vi "Lab Panel V6.00.vi"() -> ()   [LabVIEW 2017] (continued)
                    n2891 = local read "SIG LAB04-2"() -> (w5335:T2)
                    n2892 = local read "RESULT LAB04-2"() -> (w5322:bool)
                    n2893 = Bundle("FAIL LAB04-2"=w5325, "SIG LAB04-2"=w5335, "TEMP START LAB04-2"=w5334, "DISP LAB04-2"=w5331, "SET LAB04-2"=w5330, "TDMS LAB04-2"=w5333) -> (w5320:T47)  [unwired: 1 in]
                    n2894 = call "sub vi - cycle&temp fail v7.vi"("Amps Lo?"=w5332, "Input Cluster"=w5320, "SELECT"=w5329, "Amps Hi?"=w5328, "Result In"=w5322, "Panel"=u64 8) -> ("(FAIL) out"=w5324:cluster{"FAIL LO":dbl, "FAIL HI":dbl}, "(DISP) out"=w5327:T40, "T-RISE"=w5321:cluster{"T-RISE (L)":dbl, "T-RISE (N)":dbl}, "Result Out"=w5323:bool, "file error"=w5326:errorcluster)  [unwired: 9 in]
                    n2895 = local write "TEMP RISE LAB04-2"(w5321) -> ()
                    n2896 = local write "FAIL LAB04-2"(w5324) -> ()
                    n2897 = local write "DISP LAB04-2"(w5327) -> ()
                    n2898 = local write "RESULT LAB04-2"(w5323) -> ()
                    n2899 = local write "data file error"(w5326) -> ()
                  }
                }
              }
              frame #8 {
                # "LAB05-1"
                n2900 = Index Array(array=w5338, index=4) -> (element=w5341:bool)
                n2901 = Not(x=w5341) -> (.not. x?=w5339:bool)
                n2902 = And(x=w5339, y=w5337) -> (x .and. y?=w5336:bool)
                n2903 = case shown="True" w5336 {
                  tunnel: w5344 -> [_ w5358]
                  tunnel: w5342 -> [_ w5355]
                  tunnel: w5343 -> [_ w5354]
                  frame False {
                  }
                  frame True {
                    n2904 = local read "TEMP START LAB05-1"() -> (w5360:cluster{"TL":dbl, "TN":dbl})
                    n2905 = local read "FAIL LAB05-1"() -> (w5351:cluster{"LO":dbl, "HI":dbl})
                    n2906 = local read "TDMS LAB05-1"() -> (w5359:refnum<k34>)
                    n2907 = local read "SET LAB05-1"() -> (w5356:T5)
                    n2908 = local read "DISP LAB05-1"() -> (w5357:T4)
                    n2909 = local read "SIG LAB05-1"() -> (w5361:T2)
                    n2910 = local read "RESULT LAB05-1"() -> (w5348:bool)
                    n2911 = Bundle("FAIL LAB05-1"=w5351, "SIG LAB05-1"=w5361, "TEMP START LAB05-1"=w5360, "DISP LAB05-1"=w5357, "SET LAB05-1"=w5356, "TDMS LAB05-1"=w5359) -> (w5346:T48)  [unwired: 1 in]
                    n2912 = call "sub vi - cycle&temp fail v7.vi"("Amps Lo?"=w5358, "Input Cluster"=w5346, "SELECT"=w5355, "Amps Hi?"=w5354, "Result In"=w5348, "Panel"=u64 9) -> ("(FAIL) out"=w5350:cluster{"FAIL LO":dbl, "FAIL HI":dbl}, "(DISP) out"=w5353:T40, "T-RISE"=w5347:cluster{"T-RISE (L)":dbl, "T-RISE (N)":dbl}, "Result Out"=w5349:bool, "file error"=w5352:errorcluster)  [unwired: 9 in]
                    n2913 = local write "TEMP RISE LAB05-1"(w5347) -> ()
                    n2914 = local write "FAIL LAB05-1"(w5350) -> ()
                    n2915 = local write "DISP LAB05-1"(w5353) -> ()
                    n2916 = local write "RESULT LAB05-1"(w5349) -> ()
                    n2917 = local write "data file error"(w5352) -> ()
                  }
                }
              }
              frame #9 {
                # "LAB05-2"
                n2918 = Index Array(array=w5364, index=4) -> (element=w5367:bool)
                n2919 = Not(x=w5367) -> (.not. x?=w5365:bool)
                n2920 = And(x=w5365, y=w5363) -> (x .and. y?=w5362:bool)
                n2921 = case shown="True" w5362 {
                  tunnel: w5370 -> [_ w5384]
                  tunnel: w5368 -> [_ w5381]
                  tunnel: w5369 -> [_ w5380]
                  frame False {
                  }
                  frame True {
                    n2922 = local read "TEMP START LAB05-2"() -> (w5386:cluster{"TL":dbl, "TN":dbl})
                    n2923 = local read "FAIL LAB05-2"() -> (w5377:cluster{"LO":dbl, "HI":dbl})
                    n2924 = local read "TDMS LAB05-2"() -> (w5385:refnum<k34>)
                    n2925 = local read "SET LAB05-2"() -> (w5382:T5)
                    n2926 = local read "DISP LAB05-2"() -> (w5383:T4)
                    n2927 = local read "SIG LAB05-2"() -> (w5387:T2)
                    n2928 = local read "RESULT LAB05-2"() -> (w5374:bool)
                    n2929 = Bundle("FAIL LAB05-2"=w5377, "SIG LAB05-2"=w5387, "TEMP START LAB05-2"=w5386, "DISP LAB05-2"=w5383, "SET LAB05-2"=w5382, "TDMS LAB05-2"=w5385) -> (w5372:T49)  [unwired: 1 in]
                    n2930 = call "sub vi - cycle&temp fail v7.vi"("Amps Lo?"=w5384, "Input Cluster"=w5372, "SELECT"=w5381, "Amps Hi?"=w5380, "Result In"=w5374, "Panel"=u64 10) -> ("(FAIL) out"=w5376:cluster{"FAIL LO":dbl, "FAIL HI":dbl}, "(DISP) out"=w5379:T40, "T-RISE"=w5373:cluster{"T-RISE (L)":dbl, "T-RISE (N)":dbl}, "Result Out"=w5375:bool, "file error"=w5378:errorcluster)  [unwired: 9 in]
                    n2931 = local write "TEMP RISE LAB05-2"(w5373) -> ()
                    n2932 = local write "FAIL LAB05-2"(w5376) -> ()
                    n2933 = local write "DISP LAB05-2"(w5379) -> ()
                    n2934 = local write "RESULT LAB05-2"(w5375) -> ()
                    n2935 = local write "data file error"(w5378) -> ()
                  }
                }
              }
            }
            n2936 = global write "Global 1.vi" "fail count"(w5101) -> ()
          }
          frame #17 {
            # "run calibration routine"
            n2937 = case shown="True" "SET (cal)" {
              frame False {
              }
              frame True {
                n2938 = stacked-sequence {
                  seq-local: [w5389 _ _] -> [_ w5391 _]
                  frame #0 {
                    n2939 = call "CALIBRATION PASSWORD"() -> ("PASSWORD"=w5389:string)  [unwired: 17 in, 2 out]
                  }
                  frame #1 {
                    n2940 = Equal?(x=w5391, y="7777") -> (x = y?=w5390:bool)
                    n2941 = case shown="True" w5390 {
                      frame False {
                      }
                      frame True {
                        n2942 = stacked-sequence {
                          frame #0 {
                            n2943 = local read "SAMPLES"() -> (w5393:dbl)
                            n2944 = local read "AI Task2"() -> (w5394:u32)
                            n2945 = local read "AI Task1"() -> (w5395:u32)
                            n2946 = local read "AI Task0"() -> (w5396:u64)
                            n2947 = local read "Temp Test Cal"() -> (w5397:dbl)
                            n2948 = call "sub vi - calibration v2.vi"("Samples"=w5393, "Task2"=w5394, "Task1"=w5395, "Task0"=w5396, "Temp Test Cal"=w5397) -> ()  [unwired: 7 in]
                          }
                          frame #1 {
                            n2949 = call "sub vi - get calibration values v1.vi"() -> ("TEMP REF CAL"=w5399:dbl, "LAB01 (CAL)"=w5403:T15, "LAB02 (CAL)"=w5402:T16, "LAB03 (CAL)"=w5401:T15, "LAB04 (CAL)"=w5400:T15, "calibration file error out"=w5404:errorcluster, "LAB05 (CAL)"=w5398:T15)  [unwired: 9 in]
                            n2950 = local write "TEMP REF cal"(w5399) -> ()
                            n2951 = local write "cal file error out"(w5404) -> ()
                            n2952 = local write "CAL LAB04"(w5400) -> ()
                            n2953 = local write "LAB05 (CAL)"(w5398) -> ()
                            n2954 = local write "CAL LAB01"(w5403) -> ()
                            n2955 = local write "CAL LAB02"(w5402) -> ()
                            n2956 = local write "CAL LAB03"(w5401) -> ()
                          }
                        }
                      }
                    }
                  }
                  frame #2 {
                    n2957 = local write "SET (cal)"(FALSE) -> ()
                  }
                }
              }
            }
          }
          frame #18 {
            # "save certain settings to file"
            n2958 = String To Path(string="c:\\crabtree\\Set Up\\") -> (path=w5407:path)
            n2959 = Build Path(base path=w5407, name or relative path="settings.bin") -> (appended path=w5409:path)
            n2960 = Build Path(base path=w5407, name or relative path="mail.bin") -> (appended path=w5406:path)
            n2961 = Create Folder(path (use dialog)=w5407) -> (error out=w5412:errorcluster)  [unwired: 2 in, 2 out]
            n2962 = call <vilib>:"Clear Errors.vi"("error in (no error)"=w5412) -> ()  [unwired: 5 in, 2 out]
            n2963 = stacked-sequence {
              seq-local: [w5426 _] -> [_ w5439]
              tunnel: w5409 -> [_ w5440]
              tunnel: w5406 -> [_ w5438]
              frame #0 {
                n2964 = local read "Set Loop Time"() -> (w5414:T14)
                n2965 = local read "DigOutDelay"() -> (w5413:u32)
                n2966 = local read "Network Directory"() -> (w5431:path)
                n2967 = local read "C drive data root dir"() -> (w5425:path)
                n2968 = local read "RATE (Hz)"() -> (w5424:dbl)
                n2969 = local read "SAMPLES"() -> (w5423:dbl)
                n2970 = local read "Select COM port"() -> (w5422:refnum<visa-resource-name>)
                n2971 = local read "Temp Delay Lps"() -> (w5421:dbl)
                n2972 = local read "Temp Value"() -> (w5420:dbl)
                n2973 = local read "Fail Loops"() -> (w5419:dbl)
                n2974 = local read "Temp Test Cal"() -> (w5418:dbl)
                n2975 = local read "Amps Fail level"() -> (w5417:dbl)
                n2976 = local read "Mail Test File To:"() -> (w5416:string)
                n2977 = local read "Mail Test Fail"() -> (w5415:bool)
                n2978 = local read "SET LAB05-2"() -> (w5430:T5)
                n2979 = local read "SET LAB05-1"() -> (w5429:T5)
                n2980 = local read "SET LAB04-2"() -> (w5428:T5)
                n2981 = local read "SET LAB03-2"() -> (w5432:T5)
                n2982 = local read "SET LAB04-1"() -> (w5427:T5)
                n2983 = local read "SET LAB03-1"() -> (w5433:T5)
                n2984 = local read "SET LAB02-2"() -> (w5434:T5)
                n2985 = local read "SET LAB02-1"() -> (w5435:T5)
                n2986 = local read "SET LAB01-2"() -> (w5436:T5)
                n2987 = local read "SET LAB01-1"() -> (w5437:T5)
                n2988 = Bundle("SET LAB01-1"=w5437, "SET LAB01-2"=w5436, "SET LAB02-1"=w5435, "SET LAB02-2"=w5434, "SET LAB03-1"=w5433, "SET LAB03-2"=w5432, "SET LAB04-1"=w5427, "SET LAB04-2"=w5428, "SET LAB05-1"=w5429, "SET LAB05-2"=w5430, "Network Directory"=w5431, "C drive data root dir"=w5425, "RATE (Hz)"=w5424, "SAMPLES"=w5423, "Select COM port"=w5422, "Temp Delay Lps"=w5421, "Temp Value"=w5420, "Fail Loops"=w5419, "Temp Test Cal"=w5418, "Amps Fail level"=w5417, "Mail Test File To:"=w5416, "Mail Test Fail"=w5415, "Set Loop Time"=w5414, "DigOutDelay"=w5413) -> (w5426:T26)  [unwired: 1 in]
              }
              frame #1 {
                n2989 = event shown="[1] \"SET LAB01-1\", \"SET LAB01-2\", \"SET LAB02-1\", \"SET LAB02-2\", \"SET LAB03-1\", \"SET LAB03-2\", \"SET LAB04-1\", \"SET LAB04-2\", \"SET LAB05-1\", \"SET LAB05-2\", \"Network Directory\", \"C drive data root dir\", \"RATE (Hz)\", \"SAMPLES\", \"Select COM port\", \"Temp Delay Lps\", \"Temp Value\", \"Fail Loops\", \"Temp Test Cal\", \"Amps Fail level\", \"Mail Test File To:\", \"Mail Test Fail\", \"Set Loop Time\", \"DigOutDelay\": Value Change" {
                  selector: _ -> [_ _ _]
                  dyn-events: _ -> [_ _ _]
                  timeout: 0.0 -> [_ _ _]
                  tunnel: w5440 -> [_ w5442 _]
                  tunnel: w5439 -> [_ w5443 _]
                  tunnel: w5438 -> [_ _ w5454]
                  event Timeout {
                    n2990 = event-data() -> ()  [unwired: 1 in, 3 out]
                  }
                  event "Network Directory", "C drive data root dir", "RATE (Hz)", "SAMPLES", "Select COM port", "Temp Delay Lps", "Temp Value", "Fail Loops", "Temp Test Cal", "Amps Fail level", "Mail Test File To:", "Mail Test Fail", "DigOutDelay": Value Change {
                    # "Write Settings File"
                    n2991 = event-data() -> ()  [unwired: 1 in, 6 out]
                    n2992 = Open/Create/Replace File(file path (use dialog)=w5442, operation (0:open)=T19."replace or create") -> (refnum out=w5448:refnum<file>, error out=w5447:errorcluster)  [unwired: 4 in, 1 out]
                    n2993 = Write to Binary File(file (use dialog)=w5448, data=w5443, error in=w5447) -> (refnum out=w5446:refnum<file>, error out=w5445:errorcluster)  [unwired: 3 in, 1 out]
                    n2994 = Close File(refnum=w5446, error in=w5445) -> (error out=w5444:errorcluster)  [unwired: 1 out]
                    n2995 = local write "data file error"(w5444) -> ()
                  }
                  event "MAIL SETTINGS.OUT SERVER ADDRESS", "MAIL SETTINGS.FROM ACCOUNT", "MAIL SETTINGS.USER NAME", "MAIL SETTINGS.PASSWORD", "Auto Mail Send", "TO (string):": Value Change {
                    n2996 = event-data() -> ()  [unwired: 1 in, 6 out]
                    n2997 = local read "Auto Mail Send"() -> (w5451:bool)
                    n2998 = local read "MAIL SETTINGS"() -> (w5453:T7)
                    n2999 = local read "TO (string):"() -> (w5450:string)
                    n3000 = Open/Create/Replace File(file path (use dialog)=w5454, operation (0:open)=T19."replace or create") -> (refnum out=w5459:refnum<file>, error out=w5458:errorcluster)  [unwired: 4 in, 1 out]
                    n3001 = Bundle("MAIL SETTINGS"=w5453, "Auto Mail Send"=w5451, "TO (string):"=w5450) -> (w5452:T50)  [unwired: 1 in]
                    n3002 = Write to Binary File(file (use dialog)=w5459, data=w5452, error in=w5458) -> (refnum out=w5457:refnum<file>, error out=w5456:errorcluster)  [unwired: 3 in, 1 out]
                    n3003 = Close File(refnum=w5457, error in=w5456) -> (error out=w5455:errorcluster)  [unwired: 1 out]
                    n3004 = local write "data file error"(w5455) -> ()
                  }
                }
              }
            }
          }
          frame #19 {
            # "mail control"
            n3005 = local read "MAIL SETTINGS"() -> (w5476:T7)
            n3006 = local read "Auto Mail Send"() -> (w5462:bool)
            n3007 = Unbundle By Name(w5476) -> ("OUT SERVER ADDRESS"=w5475:string, "FROM ACCOUNT"=w5474:string, "TEST MAIL"=w5473:bool)
            n3008 = stacked-sequence {
              tunnel: "TO (string):" -> [_ w5515]
              tunnel: w5476 -> [w5481 w5514]
              tunnel: w5475 -> [w5480 w5513]
              tunnel: w5474 -> [w5479 w5512]
              tunnel: w5473 -> [w5478 _]
              tunnel: w5462 -> [_ w5511]
              tunnel: w5472 -> [_ w5510]
              tunnel: w5471 -> [_ w5509]
              tunnel: w5470 -> [_ w5508]
              tunnel: w5469 -> [_ w5507]
              tunnel: w5468 -> [_ w5506]
              tunnel: w5467 -> [_ w5505]
              tunnel: w5466 -> [_ w5504]
              tunnel: w5465 -> [_ w5503]
              tunnel: w5464 -> [_ w5502]
              tunnel: w5463 -> [_ w5501]
              tunnel: "TO (string):" -> [w5477 _]
              frame #0 {
                # "mail test"
                n3009 = case shown="True" w5478 {
                  tunnel: w5481 -> [_ w5485]
                  tunnel: w5477 -> [_ w5484]
                  tunnel: w5480 -> [_ w5483]
                  tunnel: w5479 -> [_ w5482]
                  frame False {
                  }
                  frame True {
                    n3010 = stacked-sequence {
                      seq-local: [_ _ w5495 _] -> [_ _ _ w5496]
                      tunnel: w5485 -> [w5488 _ _ w5500]
                      tunnel: w5484 -> [_ _ w5493 _]
                      tunnel: w5483 -> [_ _ w5491 _]
                      tunnel: w5482 -> [_ _ w5492 _]
                      frame #0 {
                        n3011 = Bundle(cluster=w5488, "TEST MAIL STATUS"="TEST START") -> (w5486:T7)  [unwired: 6 in]
                        n3012 = local write "MAIL SETTINGS"(w5486) -> ()
                      }
                      frame #1 {
                        n3013 = Wait (ms)(milliseconds to wait=500) -> ()  [unwired: 1 out]
                      }
                      frame #2 {
                        n3014 = call "Lab Send Mail Test.vi"("TO:"=w5493, "subject"="MAIL TEST FROM LAB PANEL", "from"=w5492, "out going server"=w5491, "message"="TEST MESSAGE") -> ("error out"=w5495:errorcluster)  [unwired: 10 in]
                      }
                      frame #3 {
                        n3015 = Bundle(cluster=w5500, "TEST MAIL"=FALSE, "TEST MAIL STATUS"="TEST END", "mail error"=w5496) -> (w5498:T7)  [unwired: 4 in]
                        n3016 = local write "MAIL SETTINGS"(w5498) -> ()
                      }
                    }
                  }
                }
              }
              frame #1 {
                # "mail report"
                n3017 = stacked-sequence {
                  seq-local: [_ w5558 _ _] -> [_ _ _ w5748]
                  seq-local: [_ _ w5661 _] -> [_ _ _ w5738]
                  seq-local: [w5525 _ _ _] -> [_ w5575 _ _]
                  seq-local: [w5524 _ _ _] -> [_ w5574 _ _]
                  seq-local: [w5522 _ _ _] -> [_ w5572 _ _]
                  seq-local: [w5523 _ _ _] -> [_ w5573 _ _]
                  seq-local: [w5521 _ _ _] -> [_ w5571 _ _]
                  seq-local: [w5520 _ _ _] -> [_ w5566 _ _]
                  seq-local: [w5519 _ _ _] -> [_ w5567 _ _]
                  seq-local: [w5518 _ _ _] -> [_ w5568 _ _]
                  seq-local: [w5517 _ _ _] -> [_ w5569 _ _]
                  seq-local: [w5516 _ _ _] -> [_ w5570 _ _]
                  tunnel: w5515 -> [_ _ _ w5749]
                  tunnel: w5514 -> [_ _ _ w5732]
                  tunnel: w5513 -> [_ _ _ w5746]
                  tunnel: w5512 -> [_ _ _ w5745]
                  tunnel: w5511 -> [w5556 _ _ w5740]
                  tunnel: w5510 -> [_ _ w5691 _]
                  tunnel: w5509 -> [_ _ w5688 _]
                  tunnel: w5508 -> [_ _ w5687 _]
                  tunnel: w5507 -> [_ _ w5686 _]
                  tunnel: w5506 -> [_ _ w5685 _]
                  tunnel: w5505 -> [_ _ w5684 _]
                  tunnel: w5504 -> [_ _ w5683 _]
                  tunnel: w5503 -> [_ _ w5682 _]
                  tunnel: w5502 -> [_ _ w5681 _]
                  tunnel: w5501 -> [_ _ w5680 _]
                  frame #0 {
                    n3018 = case shown="False" w5556 {
                      frame False {
                        n3019 = local write "mail control"("") -> ()
                      }
                      frame True {
                      }
                    }
                    n3020 = local read "SET LAB01-1"() -> (w5555:T5)
                    n3021 = local read "SET LAB01-2"() -> (w5554:T5)
                    n3022 = local read "SET LAB02-1"() -> (w5553:T5)
                    n3023 = local read "SET LAB02-2"() -> (w5552:T5)
                    n3024 = local read "SET LAB03-1"() -> (w5551:T5)
                    n3025 = local read "SET LAB04-1"() -> (w5549:T5)
                    n3026 = local read "SET LAB05-1"() -> (w5547:T5)
                    n3027 = local read "SET LAB03-2"() -> (w5550:T5)
                    n3028 = local read "SET LAB04-2"() -> (w5548:T5)
                    n3029 = local read "SET LAB05-2"() -> (w5546:T5)
                    n3030 = Unbundle(w5551) -> ("DESCRIPTION"=w5531:string)  [unwired: 4 out]
                    n3031 = Unbundle(w5550) -> ("DESCRIPTION"=w5530:string)  [unwired: 4 out]
                    n3032 = Unbundle(w5549) -> ("DESCRIPTION"=w5529:string)  [unwired: 4 out]
                    n3033 = Unbundle(w5546) -> ("DESCRIPTION"=w5526:string)  [unwired: 4 out]
                    n3034 = Unbundle(w5552) -> ("DESCRIPTION"=w5532:string)  [unwired: 4 out]
                    n3035 = Unbundle(w5548) -> ("DESCRIPTION"=w5528:string)  [unwired: 4 out]
                    n3036 = Unbundle(w5555) -> ("DESCRIPTION"=w5544:string)  [unwired: 4 out]
                    n3037 = Unbundle(w5553) -> ("DESCRIPTION"=w5533:string)  [unwired: 4 out]
                    n3038 = Unbundle(w5547) -> ("DESCRIPTION"=w5527:string)  [unwired: 4 out]
                    n3039 = Unbundle(w5554) -> ("DESCRIPTION"=w5534:string)  [unwired: 4 out]
                    n3040 = Concatenate Strings("[LAB05-2/", w5526) -> (w5516:string)
                    n3041 = Concatenate Strings("[LAB05-1/", w5527) -> (w5517:string)
                    n3042 = Concatenate Strings("[LAB04-2/", w5528) -> (w5518:string)
                    n3043 = Concatenate Strings("[LAB03-2/", w5530) -> (w5520:string)
                    n3044 = Concatenate Strings("[LAB04-1/", w5529) -> (w5519:string)
                    n3045 = Concatenate Strings("[LAB03-1/", w5531) -> (w5521:string)
                    n3046 = Concatenate Strings("[LAB01-2/", w5534) -> (w5524:string)
                    n3047 = Concatenate Strings("[LAB02-2/", w5532) -> (w5522:string)
                    n3048 = Concatenate Strings("[LAB01-1/", w5544) -> (w5525:string)
                    n3049 = Concatenate Strings("[LAB02-1/", w5533) -> (w5523:string)
                  }
                  frame #1 {
                    w5579 = "/"
                    w5580 = 2.0
                    n3050 = local read "DISP LAB01-1"() -> (w5660:T4)
                    n3051 = local read "DISP LAB01-2"() -> (w5659:T4)
                    n3052 = local read "DISP LAB02-1"() -> (w5658:T4)
                    n3053 = local read "DISP LAB03-2"() -> (w5655:T4)
                    n3054 = local read "DISP LAB02-2"() -> (w5657:T4)
                    n3055 = local read "DISP LAB03-1"() -> (w5656:T4)
                    n3056 = local read "DISP LAB04-2"() -> (w5653:T4)
                    n3057 = local read "DISP LAB04-1"() -> (w5654:T4)
                    n3058 = local read "DISP LAB05-1"() -> (w5652:T4)
                    n3059 = local read "DISP LAB05-2"() -> (w5651:T4)
                    n3060 = Unbundle By Name(w5660) -> ("CYCLE"=w5648:dbl, "MINS"=w5647:dbl, "STATUS"=w5644:string)
                    n3061 = Unbundle(w5659) -> ("CYCLE"=w5643:dbl, "MINS"=w5642:dbl, "STATUS"=w5639:string)
                    n3062 = Unbundle(w5658) -> ("CYCLE"=w5636:dbl, "MINS"=w5635:dbl, "STATUS"=w5634:string)
                    n3063 = Unbundle(w5655) -> ("CYCLE"=w5623:dbl, "MINS"=w5622:dbl, "STATUS"=w5619:string)
                    n3064 = Unbundle(w5656) -> ("CYCLE"=w5628:dbl, "MINS"=w5627:dbl, "STATUS"=w5624:string)
                    n3065 = Unbundle(w5657) -> ("CYCLE"=w5633:dbl, "MINS"=w5632:dbl, "STATUS"=w5629:string)
                    n3066 = Unbundle(w5654) -> ("CYCLE"=w5618:dbl, "MINS"=w5617:dbl, "STATUS"=w5614:string)
                    n3067 = Unbundle(w5653) -> ("CYCLE"=w5613:dbl, "MINS"=w5612:dbl, "STATUS"=w5609:string)
                    n3068 = Unbundle(w5652) -> ("CYCLE"=w5608:dbl, "MINS"=w5607:dbl, "STATUS"=w5604:string)
                    n3069 = Unbundle(w5651) -> ("CYCLE"=w5650:dbl, "MINS"=w5649:dbl, "STATUS"=w5601:string)
                    n3070 = Number To Decimal String(number=w5636) -> (decimal integer string=w5638:string)  [unwired: 1 in]
                    n3071 = Number To Decimal String(number=w5633) -> (decimal integer string=w5631:string)  [unwired: 1 in]
                    n3072 = Number To Decimal String(number=w5628) -> (decimal integer string=w5626:string)  [unwired: 1 in]
                    n3073 = Number To Decimal String(number=w5643) -> (decimal integer string=w5641:string)  [unwired: 1 in]
                    n3074 = Number To Decimal String(number=w5623) -> (decimal integer string=w5621:string)  [unwired: 1 in]
                    n3075 = Number To Decimal String(number=w5648) -> (decimal integer string=w5646:string)  [unwired: 1 in]
                    n3076 = Number To Decimal String(number=w5650) -> (decimal integer string=w5603:string)  [unwired: 1 in]
                    n3077 = Number To Decimal String(number=w5618) -> (decimal integer string=w5616:string)  [unwired: 1 in]
                    n3078 = Number To Decimal String(number=w5613) -> (decimal integer string=w5611:string)  [unwired: 1 in]
                    n3079 = Number To Decimal String(number=w5608) -> (decimal integer string=w5606:string)  [unwired: 1 in]
                    n3080 = Number To Fractional String(number=w5635, precision (6)=w5580) -> (F-format string=w5637:string)  [unwired: 2 in]
                    n3081 = Number To Fractional String(number=w5622, precision (6)=w5580) -> (F-format string=w5620:string)  [unwired: 2 in]
                    n3082 = Number To Fractional String(number=w5632, precision (6)=w5580) -> (F-format string=w5630:string)  [unwired: 2 in]
                    n3083 = Number To Fractional String(number=w5627, precision (6)=w5580) -> (F-format string=w5625:string)  [unwired: 2 in]
                    n3084 = Number To Fractional String(number=w5612, precision (6)=w5580) -> (F-format string=w5610:string)  [unwired: 2 in]
                    n3085 = Number To Fractional String(number=w5617, precision (6)=w5580) -> (F-format string=w5615:string)  [unwired: 2 in]
                    n3086 = Number To Fractional String(number=w5642, precision (6)=w5580) -> (F-format string=w5640:string)  [unwired: 2 in]
                    n3087 = Number To Fractional String(number=w5607, precision (6)=w5580) -> (F-format string=w5605:string)  [unwired: 2 in]
                    n3088 = Number To Fractional String(number=w5647, precision (6)=w5580) -> (F-format string=w5645:string)  [unwired: 2 in]
                    n3089 = Number To Fractional String(number=w5649, precision (6)=w5580) -> (F-format string=w5602:string)  [unwired: 2 in]
                    n3090 = Concatenate Strings(w5579, w5621, w5579, w5620, w5579, w5619) -> (w5595:string)
                    n3091 = Concatenate Strings(w5579, w5616, w5579, w5615, w5579, w5614) -> (w5594:string)
                    n3092 = Concatenate Strings(w5579, w5611, w5579, w5610, w5579, w5609) -> (w5593:string)
                    n3093 = Concatenate Strings(w5579, w5606, w5579, w5605, w5579, w5604) -> (w5592:string)
                    n3094 = Concatenate Strings(w5579, w5603, w5579, w5602, w5579, w5601) -> (w5591:string)
                    n3095 = Concatenate Strings(w5579, w5646, w5579, w5645, w5579, w5644) -> (w5600:string)
                    n3096 = Concatenate Strings(w5579, w5626, w5579, w5625, w5579, w5624) -> (w5596:string)
                    n3097 = Concatenate Strings(w5579, w5641, w5579, w5640, w5579, w5639) -> (w5599:string)
                    n3098 = Concatenate Strings(w5579, w5638, w5579, w5637, w5579, w5634) -> (w5598:string)
                    n3099 = Concatenate Strings(w5579, w5631, w5579, w5630, w5579, w5629) -> (w5597:string)
                    n3100 = Concatenate Strings("]", "\r") -> (w5576:string)
                    n3101 = Concatenate Strings(w5571, w5596, w5576) -> (w5586:string)
                    n3102 = Concatenate Strings(w5573, w5598, w5576) -> (w5588:string)
                    n3103 = Concatenate Strings(w5572, w5597, w5576) -> (w5587:string)
                    n3104 = Concatenate Strings(w5568, w5593, w5576) -> (w5583:string)
                    n3105 = Concatenate Strings(w5569, w5592, w5576) -> (w5584:string)
                    n3106 = Concatenate Strings(w5567, w5594, w5576) -> (w5582:string)
                    n3107 = Concatenate Strings(w5566, w5595, w5576) -> (w5581:string)
                    n3108 = Concatenate Strings(w5570, w5591, w5576) -> (w5585:string)
                    n3109 = Concatenate Strings(w5574, w5599, w5576) -> (w5589:string)
                    n3110 = Concatenate Strings(w5575, w5600, w5576) -> (w5590:string)
                    n3111 = Concatenate Strings(w5590, w5589, w5588, w5587, w5586, w5581, w5582, w5583, w5584, w5585) -> (w5559:string)
                    n3112 = Concatenate Strings("[PANEL/", "DESC/", "CYCLES/", "MINS/", "STATUS]", "\r", w5559) -> (w5558:string)
                    "MAIL REPORT" <- w5558
                    n3113 = global write "Global display 3.vi" "log all"(w5558) -> ()
                  }
                  frame #2 {
                    w5689 = "END"
                    n3114 = local read "mail control"() -> (w5690:string)
                    n3115 = case shown="False" w5685 {
                      tunnel: w5690 -> [w5714 _]
                      tunnel: w5689 -> [w5713 _]
                      tunnel: [w5712 FALSE] -> w5675
                      frame False {
                        n3116 = Equal?(x=w5714, y=w5713) -> (x = y?=w5712:bool)
                      }
                      frame True {
                      }
                    }
                    n3117 = case shown="False" w5691 {
                      tunnel: w5690 -> [w5730 _]
                      tunnel: w5689 -> [w5729 _]
                      tunnel: [w5728 FALSE] -> w5679
                      frame False {
                        n3118 = Equal?(x=w5730, y=w5729) -> (x = y?=w5728:bool)
                      }
                      frame True {
                      }
                    }
                    n3119 = case shown="False" w5688 {
                      tunnel: w5690 -> [w5726 _]
                      tunnel: w5689 -> [w5725 _]
                      tunnel: [w5724 FALSE] -> w5678
                      frame False {
                        n3120 = Equal?(x=w5726, y=w5725) -> (x = y?=w5724:bool)
                      }
                      frame True {
                      }
                    }
                    n3121 = case shown="False" w5686 {
                      tunnel: w5690 -> [w5718 _]
                      tunnel: w5689 -> [w5717 _]
                      tunnel: [w5716 FALSE] -> w5676
                      frame False {
                        n3122 = Equal?(x=w5718, y=w5717) -> (x = y?=w5716:bool)
                      }
                      frame True {
                      }
                    }
                    n3123 = case shown="False" w5687 {
                      tunnel: w5690 -> [w5722 _]
                      tunnel: w5689 -> [w5721 _]
                      tunnel: [w5720 FALSE] -> w5677
                      frame False {
                        n3124 = Equal?(x=w5722, y=w5721) -> (x = y?=w5720:bool)
                      }
                      frame True {
                      }
                    }
                    n3125 = Or(x=w5677, y=w5676) -> (x .or. y?=w5668:bool)
                    n3126 = Or(x=w5679, y=w5678) -> (x .or. y?=w5669:bool)
                    n3127 = Or(x=w5669, y=w5668) -> (x .or. y?=w5664:bool)
                    n3128 = case shown="False" w5681 {
                      tunnel: w5690 -> [w5698 _]
                      tunnel: w5689 -> [w5697 _]
                      tunnel: [w5696 FALSE] -> w5670
                      frame False {
                        n3129 = Equal?(x=w5698, y=w5697) -> (x = y?=w5696:bool)
                      }
                      frame True {
                      }
                    }
                    n3130 = case shown="False" w5680 {
                      tunnel: w5690 -> [w5694 _]
                      tunnel: w5689 -> [w5693 _]
                      tunnel: [w5692 FALSE] -> w5674
                      frame False {
                        n3131 = Equal?(x=w5694, y=w5693) -> (x = y?=w5692:bool)
                      }
                      frame True {
                      }
                    }
                    n3132 = case shown="False" w5682 {
                      tunnel: w5690 -> [w5702 _]
                      tunnel: w5689 -> [w5701 _]
                      tunnel: [w5700 FALSE] -> w5671
                      frame False {
                        n3133 = Equal?(x=w5702, y=w5701) -> (x = y?=w5700:bool)
                      }
                      frame True {
                      }
                    }
                    n3134 = case shown="False" w5684 {
                      tunnel: w5690 -> [w5710 _]
                      tunnel: w5689 -> [w5709 _]
                      tunnel: [w5708 FALSE] -> w5673
                      frame False {
                        n3135 = Equal?(x=w5710, y=w5709) -> (x = y?=w5708:bool)
                      }
                      frame True {
                      }
                    }
                    n3136 = case shown="False" w5683 {
                      tunnel: w5690 -> [w5706 _]
                      tunnel: w5689 -> [w5705 _]
                      tunnel: [w5704 FALSE] -> w5672
                      frame False {
                        n3137 = Equal?(x=w5706, y=w5705) -> (x = y?=w5704:bool)
                      }
                      frame True {
                      }
                    }
                    n3138 = Or(x=w5673, y=w5672) -> (x .or. y?=w5667:bool)
                    n3139 = Or(x=w5671, y=w5670) -> (x .or. y?=w5666:bool)
                    n3140 = Or(x=w5674, y=w5675) -> (x .or. y?=w5662:bool)
                    n3141 = Or(x=w5667, y=w5666) -> (x .or. y?=w5665:bool)
                    n3142 = Or(x=w5664, y=w5665) -> (x .or. y?=w5663:bool)
                    n3143 = Or(x=w5663, y=w5662) -> (x .or. y?=w5661:bool)
                  }
                  frame #3 {
                    n3144 = local read "on loops"() -> (w5744:dbl)
                    n3145 = local read "jig cycle"() -> (w5741:dbl)
                    n3146 = local read "Send Mail Now"() -> (w5735:bool)
                    n3147 = Add(x=w5744, y=5.0) -> (x+y=w5742:dbl)
                    n3148 = Equal?(x=w5741, y=w5742) -> (x = y?=w5736:bool)
                    n3149 = And(x=w5736, y=w5735) -> (x .and. y?=w5734:bool)
                    n3150 = And(x=w5740, y=w5736) -> (x .and. y?=w5739:bool)
                    n3151 = And(x=w5739, y=w5738) -> (x .and. y?=w5737:bool)
                    n3152 = Or(x=w5737, y=w5734) -> (x .or. y?=w5733:bool)
                    n3153 = case shown="True" w5733 {
                      tunnel: w5749 -> [_ w5755]
                      tunnel: w5748 -> [_ w5754]
                      tunnel: "Lab Panel Test Status" -> [_ w5753]
                      tunnel: w5746 -> [_ w5752]
                      tunnel: w5745 -> [_ w5751]
                      tunnel: w5732 -> [_ w5750]
                      frame False {
                      }
                      frame True {
                        n3154 = stacked-sequence {
                          tunnel: w5755 -> [w5764 _]
                          tunnel: w5754 -> [w5763 _]
                          tunnel: w5753 -> [w5762 _]
                          tunnel: w5752 -> [w5761 _]
                          tunnel: w5751 -> [w5760 _]
                          tunnel: w5750 -> [w5759 _]
                          frame #0 {
                            n3155 = call "Lab Send Mail Test.vi"("TO:"=w5764, "subject"=w5762, "Info"="Test station status report", "from"=w5760, "out going server"=w5761, "message"=w5763) -> ("error out"=w5758:errorcluster)  [unwired: 9 in]
                            n3156 = Bundle(cluster=w5759, "mail error"=w5758) -> (w5757:T7)  [unwired: 6 in]
                            n3157 = local write "MAIL SETTINGS"(w5757) -> ()
                          }
                          frame #1 {
                            n3158 = local write "mail control"("") -> ()
                            n3159 = local write "Send Mail Now"(FALSE) -> ()
                          }
                        }
                      }
                    }
                  }
                }
              }
            }
          }
          frame #20 {
            # "save jig cycle values once all run switches are off"
            n3160 = stacked-sequence {
              tunnel: w5776 -> [_ w5805]
              tunnel: w5775 -> [_ w5804]
              tunnel: w5774 -> [_ w5803]
              tunnel: w5773 -> [_ w5802]
              tunnel: w5772 -> [_ w5801]
              tunnel: w5771 -> [_ w5800]
              tunnel: w5770 -> [_ w5799]
              tunnel: w5769 -> [_ w5798]
              tunnel: w5768 -> [_ w5797]
              tunnel: w5767 -> [_ w5796]
              frame #0 {
              }
              frame #1 {
                n3161 = Not(x=w5796) -> (.not. x?=w5779:bool)
                n3162 = Not(x=w5804) -> (.not. x?=w5794:bool)
                n3163 = Not(x=w5801) -> (.not. x?=w5789:bool)
                n3164 = Not(x=w5799) -> (.not. x?=w5785:bool)
                n3165 = Not(x=w5797) -> (.not. x?=w5781:bool)
                n3166 = Not(x=w5805) -> (.not. x?=w5795:bool)
                n3167 = Not(x=w5803) -> (.not. x?=w5793:bool)
                n3168 = Not(x=w5800) -> (.not. x?=w5787:bool)
                n3169 = Not(x=w5802) -> (.not. x?=w5791:bool)
                n3170 = Not(x=w5798) -> (.not. x?=w5783:bool)
                n3171 = local read "Save JC"() -> (w5807:bool)
                n3172 = And(x=w5795, y=w5794) -> (x .and. y?=w5792:bool)
                n3173 = And(x=w5792, y=w5793) -> (x .and. y?=w5790:bool)
                n3174 = And(x=w5790, y=w5791) -> (x .and. y?=w5788:bool)
                n3175 = And(x=w5788, y=w5789) -> (x .and. y?=w5786:bool)
                n3176 = And(x=w5786, y=w5787) -> (x .and. y?=w5784:bool)
                n3177 = And(x=w5784, y=w5785) -> (x .and. y?=w5782:bool)
                n3178 = And(x=w5782, y=w5783) -> (x .and. y?=w5780:bool)
                n3179 = And(x=w5780, y=w5781) -> (x .and. y?=w5778:bool)
                n3180 = And(x=w5778, y=w5779) -> (x .and. y?=w5777:bool)
                n3181 = And(x=w5777, y=w5807) -> (x .and. y?=w5806:bool)
                n3182 = case shown="True" w5806 {
                  tunnel: w5777 -> [w5808 _]
                  frame False {
                    n3183 = case shown="False" w5808 {
                      frame False {
                        n3184 = local write "Save JC"(TRUE) -> ()
                      }
                      frame True {
                      }
                    }
                  }
                  frame True {
                    n3185 = stacked-sequence {
                      frame #0 {
                        n3186 = String To Path(string="c:\\crabtree\\Jig Cycles\\") -> (path=w5820:path)
                        n3187 = Build Path(base path=w5820, name or relative path="jigcycles.bin") -> (appended path=w5818:path)
                        n3188 = Create Folder(path (use dialog)=w5820) -> (error out=w5822:errorcluster)  [unwired: 2 in, 2 out]
                        n3189 = local read "JIG RELAY CYCLES"() -> (w5812:T8)
                        n3190 = call <vilib>:"Clear Errors.vi"("error in (no error)"=w5822) -> ()  [unwired: 5 in, 2 out]
                        n3191 = local write "Save JC"(FALSE) -> ()
                        n3192 = Open/Create/Replace File(file path (use dialog)=w5818, operation (0:open)=T19."replace or create") -> (refnum out=w5816:refnum<file>, error out=w5817:errorcluster)  [unwired: 4 in, 1 out]
                        n3193 = Write to Binary File(file (use dialog)=w5816, data=w5812, error in=w5817) -> (refnum out=w5815:refnum<file>, error out=w5814:errorcluster)  [unwired: 3 in, 1 out]
                        n3194 = Close File(refnum=w5815, error in=w5814) -> (error out=w5813:errorcluster)  [unwired: 1 out]
                        n3195 = local write "data file error"(w5813) -> ()
                      }
                      frame #1 {
                        n3196 = local read "JIG RELAY CYCLES"() -> (w5845:T8)
                        n3197 = Unbundle By Name(w5845) -> ("LAB01-1"=w5840:dbl, "LAB01-2"=w5839:dbl, "LAB02-1"=w5837:dbl, "LAB02-2"=w5836:dbl, "LAB03-1"=w5834:dbl, "LAB03-2"=w5831:dbl, "LAB04-1"=w5830:dbl, "LAB04-2"=w5828:dbl, "LAB05-1"=w5826:dbl, "LAB05-2"=w5824:dbl)
                        n3198 = stacked-sequence {
                          tunnel: w5840 -> [w5848 _ _ _ _ _ _ _ _ _]
                          tunnel: 1000000 -> [w5851 w5861 w5871 w5881 w5891 w5901 w5911 w5921 w5931 w5941]
                          tunnel: [w5849 _ _ _ _ _ _ _ _ _] -> w5843
                          tunnel: "TEST STATION HAS REACHED 1 MILLION CYCLES, REPLACE  CONTROL RELAYS" -> [w5847 w5859 w5869 w5879 w5889 w5899 w5909 w5919 w5929 w5939]
                          tunnel: [_ w5858 _ _ _ _ _ _ _ _] -> w5841
                          tunnel: w5839 -> [_ w5857 _ _ _ _ _ _ _ _]
                          tunnel: [_ _ w5868 _ _ _ _ _ _ _] -> w5838
                          tunnel: w5837 -> [_ _ w5867 _ _ _ _ _ _ _]
                          tunnel: w5836 -> [_ _ _ w5878 _ _ _ _ _ _]
                          tunnel: [_ _ _ w5877 _ _ _ _ _ _] -> w5835
                          tunnel: w5834 -> [_ _ _ _ w5888 _ _ _ _ _]
                          tunnel: [_ _ _ _ w5887 _ _ _ _ _] -> w5833
                          tunnel: [_ _ _ _ _ w5898 _ _ _ _] -> w5832
                          tunnel: w5831 -> [_ _ _ _ _ w5897 _ _ _ _]
                          tunnel: w5830 -> [_ _ _ _ _ _ w5908 _ _ _]
                          tunnel: [_ _ _ _ _ _ w5907 _ _ _] -> w5829
                          tunnel: w5828 -> [_ _ _ _ _ _ _ w5918 _ _]
                          tunnel: [_ _ _ _ _ _ _ w5917 _ _] -> w5827
                          tunnel: w5826 -> [_ _ _ _ _ _ _ _ w5928 _]
                          tunnel: [_ _ _ _ _ _ _ _ w5927 _] -> w5825
                          tunnel: w5824 -> [_ _ _ _ _ _ _ _ _ w5938]
                          tunnel: [_ _ _ _ _ _ _ _ _ w5937] -> w5823
                          frame #0 {
                            n3199 = Greater?(x=w5848, y=w5851) -> (0:w5850:bool)
                            n3200 = case shown="True" w5850 {
                              tunnel: [w5852 0] -> w5849
                              tunnel: w5848 -> [w5852 _]
                              tunnel: w5847 -> [_ w5853]
                              frame False {
                              }
                              frame True {
                                n3201 = Concatenate Strings("LA01-1 ", w5853) -> (w5856:string)
                                n3202 = One Button Dialog(message=w5856) -> ()  [unwired: 1 in, 1 out]
                              }
                            }
                          }
                          frame #1 {
                            n3203 = Greater?(x=w5857, y=w5861) -> (0:w5860:bool)
                            n3204 = case shown="True" w5860 {
                              tunnel: [w5862 0] -> w5858
                              tunnel: w5857 -> [w5862 _]
                              tunnel: w5859 -> [_ w5863]
                              frame False {
                              }
                              frame True {
                                n3205 = Concatenate Strings("LA01-2 ", w5863) -> (w5866:string)
                                n3206 = One Button Dialog(message=w5866) -> ()  [unwired: 1 in, 1 out]
                              }
                            }
                          }
                          frame #2 {
                            n3207 = Greater?(x=w5867, y=w5871) -> (0:w5870:bool)
                            n3208 = case shown="True" w5870 {
                              tunnel: [w5872 0] -> w5868
                              tunnel: w5867 -> [w5872 _]
                              tunnel: w5869 -> [_ w5873]
                              frame False {
                              }
                              frame True {
                                n3209 = Concatenate Strings("LA02-1 ", w5873) -> (w5876:string)
                                n3210 = One Button Dialog(message=w5876) -> ()  [unwired: 1 in, 1 out]
                              }
                            }
                          }
                          frame #3 {
                            n3211 = Greater?(x=w5878, y=w5881) -> (0:w5880:bool)
                            n3212 = case shown="True" w5880 {
                              tunnel: [w5882 0] -> w5877
                              tunnel: w5878 -> [w5882 _]
                              tunnel: w5879 -> [_ w5883]
                              frame False {
                              }
                              frame True {
                                n3213 = Concatenate Strings("LA02-2 ", w5883) -> (w5886:string)
                                n3214 = One Button Dialog(message=w5886) -> ()  [unwired: 1 in, 1 out]
                              }
                            }
                          }
                          frame #4 {
                            n3215 = Greater?(x=w5888, y=w5891) -> (0:w5890:bool)
                            n3216 = case shown="True" w5890 {
                              tunnel: [w5892 0] -> w5887
                              tunnel: w5888 -> [w5892 _]
                              tunnel: w5889 -> [_ w5893]
                              frame False {
                              }
                              frame True {
                                n3217 = Concatenate Strings("LA03-1 ", w5893) -> (w5896:string)
                                n3218 = One Button Dialog(message=w5896) -> ()  [unwired: 1 in, 1 out]
                              }
                            }
                          }
                          frame #5 {
                            n3219 = Greater?(x=w5897, y=w5901) -> (0:w5900:bool)
                            n3220 = case shown="True" w5900 {
                              tunnel: [w5902 0] -> w5898
                              tunnel: w5897 -> [w5902 _]
                              tunnel: w5899 -> [_ w5903]
                              frame False {
                              }
                              frame True {
                                n3221 = Concatenate Strings("LA03-2 ", w5903) -> (w5906:string)
                                n3222 = One Button Dialog(message=w5906) -> ()  [unwired: 1 in, 1 out]
                              }
                            }
                          }
                          frame #6 {
                            n3223 = Greater?(x=w5908, y=w5911) -> (0:w5910:bool)
                            n3224 = case shown="True" w5910 {
                              tunnel: [w5912 0] -> w5907
                              tunnel: w5908 -> [w5912 _]
                              tunnel: w5909 -> [_ w5913]
                              frame False {
                              }
                              frame True {
                                n3225 = Concatenate Strings("LA04-1 ", w5913) -> (w5916:string)
                                n3226 = One Button Dialog(message=w5916) -> ()  [unwired: 1 in, 1 out]
                              }
                            }
                          }
                          frame #7 {
                            n3227 = Greater?(x=w5918, y=w5921) -> (0:w5920:bool)
                            n3228 = case shown="True" w5920 {
                              tunnel: [w5922 0] -> w5917
                              tunnel: w5918 -> [w5922 _]
                              tunnel: w5919 -> [_ w5923]
                              frame False {
                              }
                              frame True {
                                n3229 = Concatenate Strings("LA04-2 ", w5923) -> (w5926:string)
                                n3230 = One Button Dialog(message=w5926) -> ()  [unwired: 1 in, 1 out]
                              }
                            }
                          }
                          frame #8 {
                            n3231 = Greater?(x=w5928, y=w5931) -> (0:w5930:bool)
                            n3232 = case shown="True" w5930 {
                              tunnel: [w5932 0] -> w5927
                              tunnel: w5928 -> [w5932 _]
                              tunnel: w5929 -> [_ w5933]
                              frame False {
                              }
                              frame True {
                                n3233 = Concatenate Strings("LA05-1 ", w5933) -> (w5936:string)
                                n3234 = One Button Dialog(message=w5936) -> ()  [unwired: 1 in, 1 out]
                              }
                            }
                          }
                          frame #9 {
                            n3235 = Greater?(x=w5938, y=w5941) -> (0:w5940:bool)
                            n3236 = case shown="True" w5940 {
                              tunnel: [w5942 0] -> w5937
                              tunnel: w5938 -> [w5942 _]
                              tunnel: w5939 -> [_ w5943]
                              frame False {
                              }
                              frame True {
                                n3237 = Concatenate Strings("LA05-2 ", w5943) -> (w5946:string)
                                n3238 = One Button Dialog(message=w5946) -> ()  [unwired: 1 in, 1 out]
                              }
                            }
                          }
                        }
                        n3239 = Bundle By Name(cluster=w5845, "LAB01-1"=w5843, "LAB01-2"=w5841, "LAB02-1"=w5838, "LAB02-2"=w5835, "LAB03-1"=w5833, "LAB03-2"=w5832, "LAB04-1"=w5829, "LAB04-2"=w5827, "LAB05-1"=w5825, "LAB05-2"=w5823) -> (w5844:T8)
                        n3240 = local write "JIG RELAY CYCLES"(w5844) -> ()
                      }
                    }
                  }
                }
              }
            }
          }
          frame #21 {
            # "get temperature values"
            n3241 = local read "DAQ Simulate"() -> (w5959:bool)
            n3242 = local read "Temp Test Cal"() -> (w5956:dbl)
            n3243 = stacked-sequence {
              seq-local: [_ w5966 _] -> [_ _ w6013]
              tunnel: w5959 -> [_ _ w6026]
              tunnel: T15 {"1  (A) cal"=1.0, "1 (V) cal"=1.0, "1 (PF) cal"=1.0, "1 (TL) cal"=1.0, "1 (TN) cal"=1.0, "2 (A) cal"=1.0, "2 (V) cal"=1.0, "2 (PF) cal"=1.0, "2 (TL) cal"=1.0, "2 (TN) cal"=1.0} ("CAL LAB01") -> [_ _ w6025]
              tunnel: w5957 -> [_ _ w6024]
              tunnel: w5956 -> [_ _ w6023]
              tunnel: w5955 -> [_ _ w6022]
              tunnel: w5954 -> [_ _ w6021]
              tunnel: w5953 -> [_ _ w6020]
              tunnel: w5952 -> [_ _ w6019]
              tunnel: w5951 -> [_ _ w6018]
              tunnel: w5950 -> [_ _ w6017]
              tunnel: w5949 -> [_ _ w6016]
              tunnel: w5948 -> [_ _ w6015]
              tunnel: w5947 -> [_ _ w6014]
              frame #0 {
                n3244 = case shown="True" "Open Com Port" {
                  frame False {
                  }
                  frame True {
                    n3245 = local read "Select COM port"() -> (w5964:refnum<visa-resource-name>)
